vi "caseNumSat.vi"(0 "emptyVarCorrArr":dbl[](array[numeric]), 1 "signalArrCDB":cdb[](array[numeric]), 2 "iFreq":dbl, 3 "Freq min":dbl, 4 "Freq cell":dbl, 5 "SampTimeArr":dbl[](array[numeric]), 6 "PSPcodeL1C/A":dbl[](array[numeric]), 7 "PSPcodeL1C/AIndex":dbl[](array[numeric]), 8 "emptyCorrArr":dbl[][](array[numeric]), 10 "numCellFreq":i32, 11 "codeFreqDivAdcFreq":dbl, 12 "timeAccumAcq":dbl, 13 "codeLength":dbl, 14 "timeStep":dbl, 15 "isThisNumTry":bool) -> (18 "mean":dbl, 20 "cn0Est":dbl, 21 "ampCorr":dbl, 22 "varCorr":dbl, 23 "cellFreqEst":dbl, 24 "cellDelayEst":dbl, 25 "dopEst":dbl, 26 "codePhase":dbl)   [LabVIEW 2020]
uses:
  <vilib>/Analysis/2dsp.llb/Real FFT.vi
  <vilib>/Analysis/NI_AALPro.lvlib
  <vilib>/Analysis/NI_AALBase.lvlib
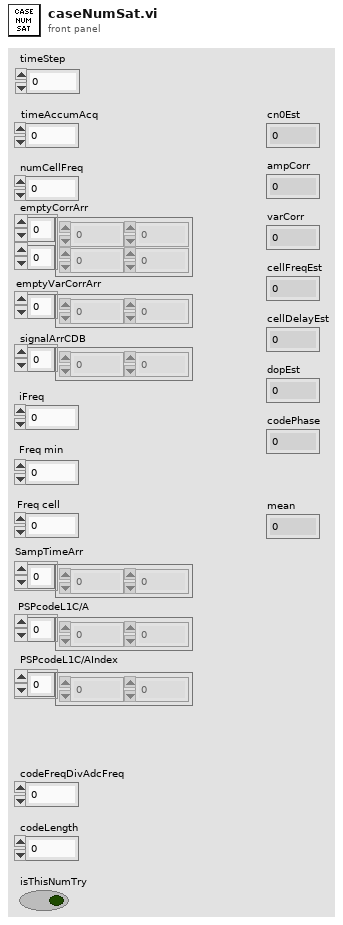
[diagram p1: front panel]
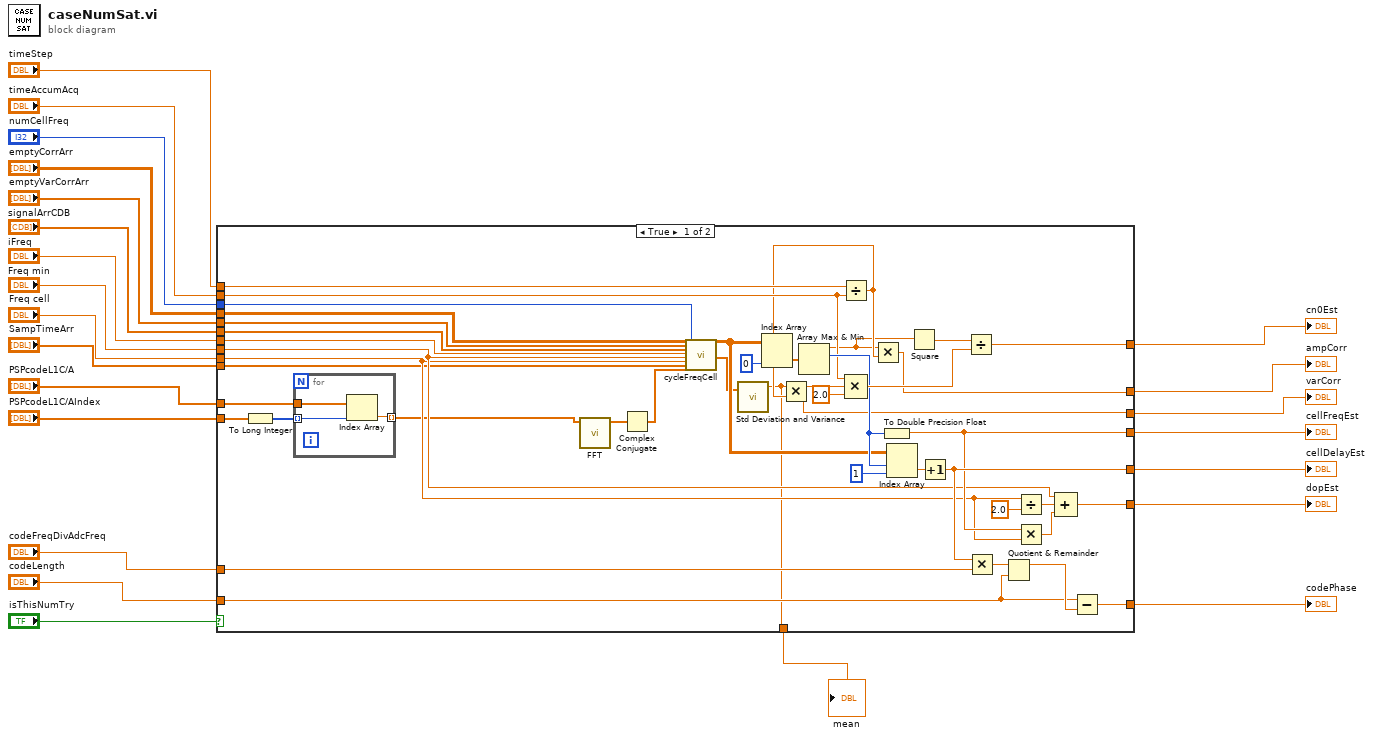
[diagram p0: block diagram]
diagram:
  n1 = case shown="True" "isThisNumTry" {
    tunnel: "PSPcodeL1C/AIndex" -> [w44 _]
    tunnel: "emptyCorrArr" -> [w42 _]
    tunnel: "numCellFreq" -> [w43 _]
    tunnel: "iFreq" -> [w35 _]
    tunnel: "SampTimeArr" -> [w39 _]
    tunnel: "signalArrCDB" -> [w36 _]
    tunnel: [w27 _] -> w7
    tunnel: [w28 _] -> w8
    tunnel: "Freq cell" -> [w40 _]
    tunnel: "Freq min" -> [w41 _]
    tunnel: [w66 _] -> w4
    tunnel: [w65 _] -> w5
    tunnel: "codeFreqDivAdcFreq" -> [w45 _]
    tunnel: "codeLength" -> [w46 _]
    tunnel: [w64 _] -> w6
    tunnel: [w63 _] -> w9
    tunnel: "timeAccumAcq" -> [w34 _]
    tunnel: [w62 _] -> w3
    tunnel: "PSPcodeL1C/A" -> [w47 _]
    tunnel: "emptyVarCorrArr" -> [w37 _]
    tunnel: "timeStep" -> [w33 _]
    tunnel: [w24 _] -> w1
    frame True {
      n2 = To Long Integer(number=w44) -> (32bit integer=w61:i32[])
      n3 = for {
        tunnel: w61 -> [w68] mode=indexing
        tunnel: w47 -> [w69]
        tunnel: [w67] -> w25 mode=indexing
        n4 = Index Array(array=w69, index=w68) -> (element=w67:dbl)
      }
      n5 = call-poly <vilib>:"FFT.vi"("X"=w25) -> ("FFT {X}"=w60:cdb[])  [unwired: 9 in, 1 out]
      n6 = Complex Conjugate(1:w60) -> (0:w38:cdb[])
      n7 = call "cycleFreqCell.vi"("emptyCorrArr"=w42, "emptyVarCorArr"=w37, "signalArrayCDB"=w36, "iFreq"=w35, "Freq min"=w41, "Freq cell"=w40, "sampTime Array"=w39, "fftCodeRefConj"=w38, "numCellFreq"=w43) -> ("corrArr"=w30:dbl[][], "ArrVarCor"=w29:dbl[])  [unwired: 16 in, 1 out]
      n8 = call <vilib>:"Std Deviation and Variance.vi"("X"=w29) -> ("mean"=w24:dbl)  [unwired: 1 in, 2 out]
      n9 = Index Array(array=w30, index (col)=0 ("disabled index (col)")) -> (element=w57:dbl[])  [unwired: 1 in]
      n10 = Array Max & Min(array=w57) -> (max value=w26:dbl, max index (indices)=w51:i32)  [unwired: 2 out]
      n11 = Divide(x=w33, y=w34) -> (x/y=w32:dbl)
      n12 = Multiply(x=w24, y=w32) -> (x*y=w27:dbl)
      n13 = Compound Arithmetic op=MULTIPLY(w34, w24, 2.0 ("value")) -> (w56:dbl)
      n14 = Multiply(x=w26, y=w32) -> (x*y=w28:dbl)
      n15 = To Double Precision Float(number=w51) -> (double precision float=w64:dbl)
      n16 = Index Array(array=w30, index (row)=w51, index (col)=1 ("disabled index (col)")) -> (element=w54:dbl)
      n17 = Square(x=w26) -> (x^2=w31:dbl)
      n18 = Increment(x=w54) -> (x+1=w65:dbl)
      n19 = Divide(x=w31, y=w56) -> (x/y=w63:dbl)
      n20 = Multiply(x=w65, y=w45) -> (x*y=w49:dbl)
      n21 = Quotient & Remainder(x=w49, y=w46) -> (x-y*floor(x/y)=w48:dbl)  [unwired: 1 out]
      n22 = Divide(x=w40, y=2.0) -> (x/y=w52:dbl)
      n23 = Multiply(x=w64, y=w40) -> (x*y=w50:dbl)
      n24 = Compound Arithmetic op=ADD(w41, w52, w50) -> (w66:dbl)
      n25 = Subtract(x=w46, y=w48) -> (x-y=w62:dbl)
    }
    frame False {
    }
  }
  "cn0Est" <- w9
  "ampCorr" <- w8
  "varCorr" <- w7
  "cellFreqEst" <- w6
  "cellDelayEst" <- w5
  "dopEst" <- w4
  "codePhase" <- w3
  "mean" <- w1
